vi "OOK_Modulation.vi"(10 "upsampling number":i32, 11 "input bit stream":i8[](array[numeric])) -> (3 "output bit stream":i8[](array[numeric]))   [LabVIEW 2014]
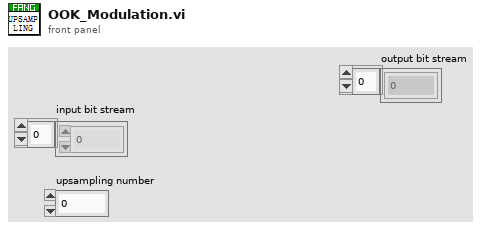
[diagram p1: front panel]
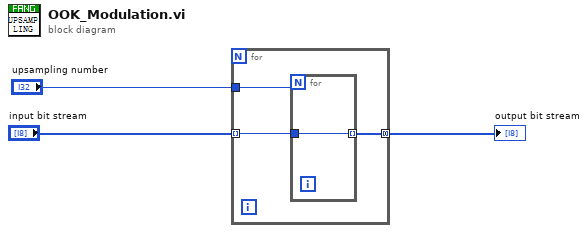
[diagram p0: block diagram]
diagram:
  n1 = for {
    tunnel: "input bit stream" -> [w5] mode=indexing
    tunnel: "upsampling number" -> [w6]
    tunnel: [w4] -> w1 mode=concatenating
    n2 = for {
      N: w6 -> [_]
      tunnel: w5 -> [w7]
      tunnel: [w7] -> w4 mode=indexing
    }
  }
  "output bit stream" <- w1
